vi "testParseStateQueueWarning_2024.vi"(8 "error in (no error)":errorcluster, 11 "testStateMachineUtilities in":refnum<class "testStateMachineUtilities.lvclass">) -> (0 "error out":errorcluster, 3 "testStateMachineUtilities out":refnum<class "testStateMachineUtilities.lvclass">)   [LabVIEW 2013, in "testStateMachineUtilities.lvclass"]
uses:
  testStateMachineUtilities.lvclass
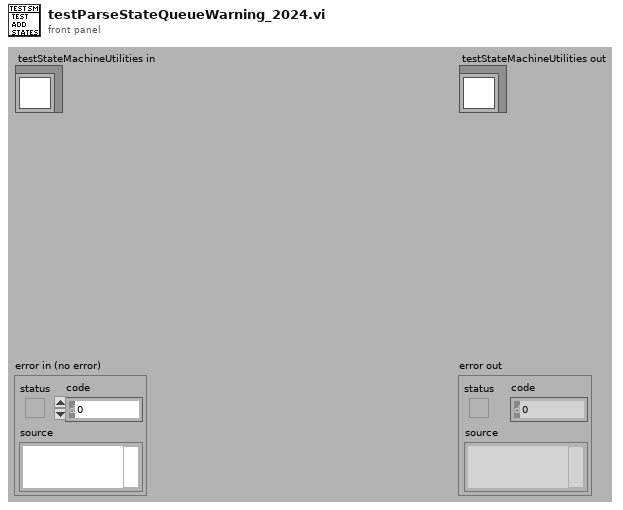
[diagram p1: front panel]
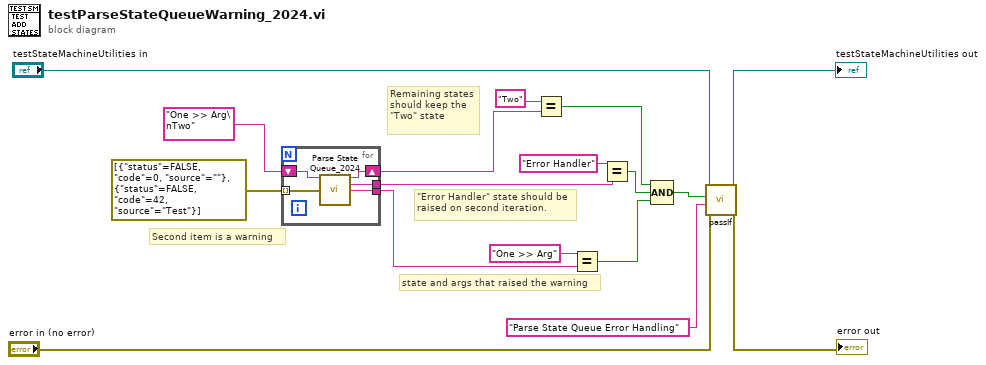
[diagram p0: block diagram]
diagram:
  # "Second item is a warning"
  # "state and args that raised the warning"
  # "\"Error Handler\" state should be raised on second iteration."
  # "Remaining states should keep the \"Two\" state"
  n1 = for {
    tunnel: errorcluster[] [{"status"=FALSE, "code"=0, "source"=""}, {"status"=FALSE, "code"=42, "source"="Test"}] -> [w22] mode=indexing
    tunnel: [w20] -> w3
    tunnel: [w19] -> w11
    shift-right: [w18] -> w6
    shift-left: "One >> Arg\nTwo" ("State Queue") -> [w21]
    n2 = call "Parse State Queue_2024.vi"("State Queue"=w21, "Error In (no error)"=w22) -> ("Remaining States"=w18:string, "Current State"=w19:string, "Arguments"=w20:string)  [unwired: 11 in]
  }
  n3 = Equal?(x="Two" ("State Queue"), y=w6) -> (x = y?=w1:bool)
  n4 = Equal?(x="One >> Arg", y=w3) -> (x = y?=w2:bool)
  n5 = Equal?(x="Error Handler", y=w11) -> (x = y?=w10:bool)
  n6 = Compound Arithmetic op=AND(w1, w10, w2) -> (w9:bool)
  n7 = call-dynamic "passIf.vi"("error in (no error)"="error in (no error)", "message (\"\")"="Parse State Queue Error Handling", "pass"=w9, "TestCase in"="testStateMachineUtilities in") -> ("error out"=→"error out":errorcluster, "TestCase out"=→"testStateMachineUtilities out":refnum<class "testStateMachineUtilities.lvclass">)  [unwired: 6 in]
